vi "NI VeriStand - Deploy UDP Channel Streaming Session.vi"(8 "error in (no error)":errorcluster, 11 "UDPChannelStreamSession in":T1) -> (0 "error out":errorcluster, 1 "Packet IDs":i32[](array[numeric]), 2 "Channel IDs":i32[](array[numeric]), 3 "UDPChannelStreamSession out":T1, 4 "Max Packet Size":i32, 5 "Port":u16, 7 "UDP Multicast Address":string)   [LabVIEW 2020, in "NI_VS Workspace ExecutionAPI.lvlib"]
doc: "Deploys a UDP channel streaming session that you open with the Open UDP Channel Streaming Session VI. This VI returns data that you can use with the LabVIEW UDP VI and functions to read data from the channels."
uses:
  <vilib>/NI VeriStand/Execution/Workspace/NI_VS Workspace ExecutionAPI.lvlib
  <vilib>/NI VeriStand/Execution/Workspace/UDPChannelStreamSession.ctl
  NationalInstruments.VeriStand.ClientAPI
  NationalInstruments.VeriStand
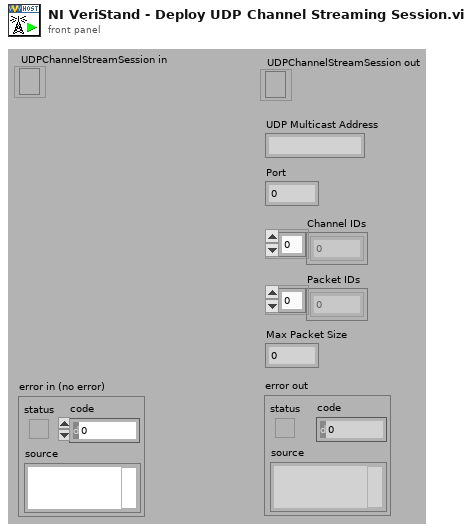
[diagram p1: front panel]
types:
  T1 = typedef "NI_VS Workspace ExecutionAPI.lvlib/UDPChannelStreamSession.ctl" = refnum<k24>
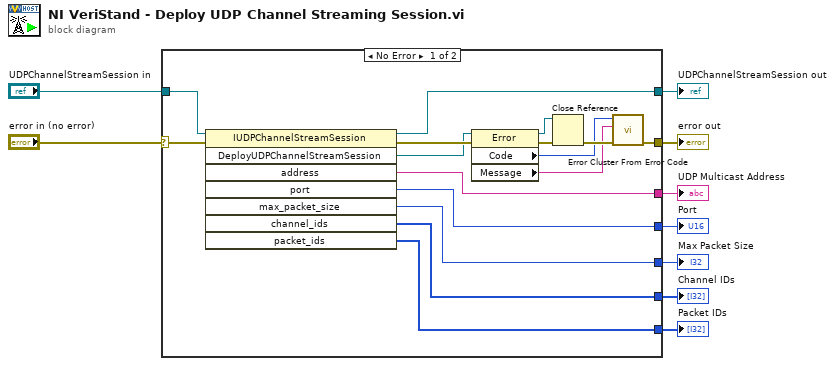
[diagram p0: block diagram]
diagram:
  n1 = case shown="No Error" "error in (no error)" {
    selector: "error in (no error)" -> [w25 w27]
    tunnel: [w17 w27] -> w9
    tunnel: "UDPChannelStreamSession in" -> [w24 w26]
    tunnel: [w23 w26] -> w6
    tunnel: [w22 _] -> w5
    tunnel: [w21 _] -> w4
    tunnel: [w20 _] -> w3
    tunnel: [w19 _] -> w2
    tunnel: [w18 _] -> w1
    frame No Error {
      n2 = invoke class="IUDPChannelStreamSession" method="DeployUDPChannelStreamSession"(reference=w24, error in=w25) -> (reference out=w23:T1, error out=w16:errorcluster, "DeployUDPChannelStreamSession"=w14:refnum<k24>, "address"=w18:string, "port"=w19:u16, "max_packet_size"=w20:i32, "channel_ids"=w21:i32[], "packet_ids"=w22:i32[])  [unwired: 6 in]
      n3 = property class="Error"(reference=w14, error in=w16) -> (reference out=w13:refnum<k24>, error out=w15:errorcluster, "Code"=w11:u32, "Message"=w10:string)
      n4 = Close Reference(reference=w13, error in (no error)=w15) -> (error out=w12:errorcluster)
      n5 = call <vilib>:"Error Cluster From Error Code.vi"("error in (no error)"=w12, "error message (\"\")"=w10, "error code (0)"=w11) -> ("error out"=w17:errorcluster)  [unwired: 6 in]
    }
    frame Error {
    }
  }
  "UDPChannelStreamSession out" <- w6
  "error out" <- w9
  "UDP Multicast Address" <- w1
  "Port" <- w2
  "Max Packet Size" <- w3
  "Channel IDs" <- w4
  "Packet IDs" <- w5
